vi "Configure Dialog.vi"(8 "error in (no error)":errorcluster, 11 "Create Arbitrary Waveform [ARB] Msg in":refnum<class "Create Arbitrary Waveform [ARB] Msg.lvclass">) -> (0 "error out":errorcluster, 2 "Ok?":bool, 3 "Create Arbitrary Waveform [ARB] Msg out":refnum<class "Create Arbitrary Waveform [ARB] Msg.lvclass">)   [LabVIEW 2014, in "CS++Fgen.lvlib" / "Create Arbitrary Waveform [ARB] Msg.lvclass"]
uses:
  Create Arbitrary Waveform [ARB] Msg.lvclass
  Create Arbitrary Waveform [ARB] Msg.lvclass/Create Arbitrary Waveform [ARB] Msg.ctl
panel:
  in  "waveform data array (empty)":dbl[](array[numeric]) caption="Waveform Data Array"
  in  "OK Button":bool
  in  "Cancel Button":bool
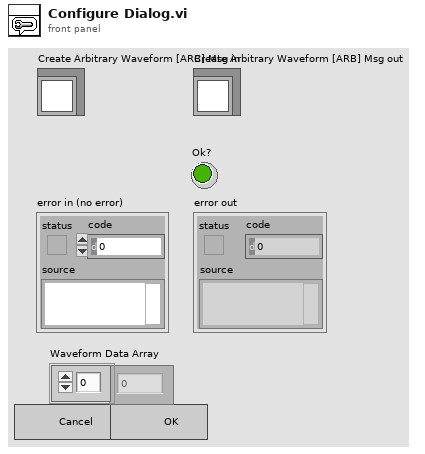
[diagram p1: front panel]
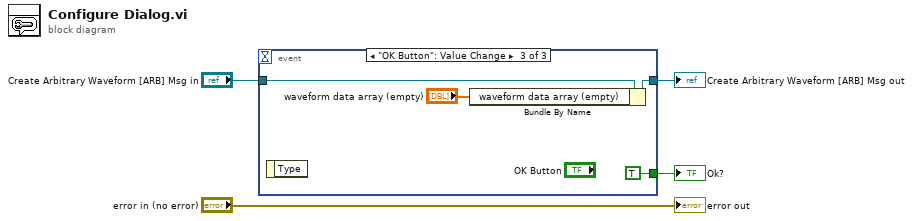
[diagram p0: block diagram]
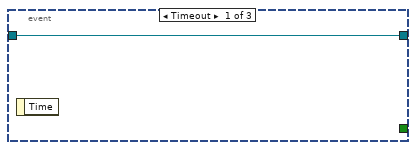
[diagram p2: hidden frame]
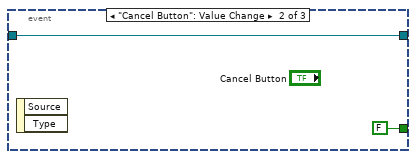
[diagram p3: hidden frame]
diagram:
  n1 = event shown="[2] \"OK Button\": Value Change" {
    selector: _ -> [_ _ _]
    dyn-events: _ -> [_ _ _]
    timeout: _ -> [_ _ _]
    tunnel: [w5 w7 w9] -> w3
    tunnel: "Create Arbitrary Waveform [ARB] Msg in" -> [w5 w7 w11]
    tunnel: [_ FALSE TRUE] -> w1
    event Timeout {
      n2 = event-data() -> ()  [unwired: 1 in, 1 out]
    }
    event "Cancel Button": Value Change {
      n3 = event-data() -> ()  [unwired: 1 in, 2 out]
    }
    event "OK Button": Value Change {
      n4 = event-data() -> ()  [unwired: 1 in, 1 out]
      n5 = Bundle By Name(cluster=w11, "waveform data array (empty)"="waveform data array (empty)") -> (w9:refnum<class "Create Arbitrary Waveform [ARB] Msg.lvclass">)
    }
  }
  "Create Arbitrary Waveform [ARB] Msg out" <- w3
  "Ok?" <- w1
  "error out" <- "error in (no error)"
